vi "PicoScope6000aGetValuesOverlapped.vi"(5 "Segment Range":T1 {"toSegmentIndex" format="%.4p"; "fromSegmentIndex" format="%.4p"}, 7 "Buffer and Transfer Settings":T2 {"Down-Sample Mode" items=["None", "Aggregate", "Decimate", "Average"]; "Down Sample Ratio" step=1; "Samples" format="%_6p"}, 8 "error in (no error)":errorcluster, 11 "handle in":i16) -> (0 "error out":errorcluster, 3 "handle out":i16, 4 "overflow":i16[](array[numeric]) format="%10b", 6 "noOfSamples":u64)   [LabVIEW 2009]
doc: "Calls ps6000aGetValues"
uses:
  ps6000a.dll
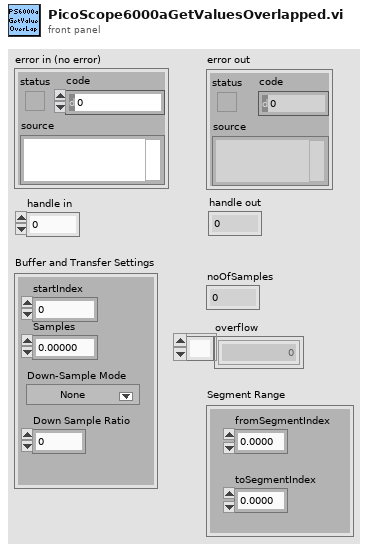
[diagram p1: front panel]
types:
  T1 = cluster{"fromSegmentIndex":u64, "toSegmentIndex":u64}
  T2 = cluster{"startIndex":u64, "Samples":u64, "Down Sample Ratio":u64, "Down-Sample Mode":u32}
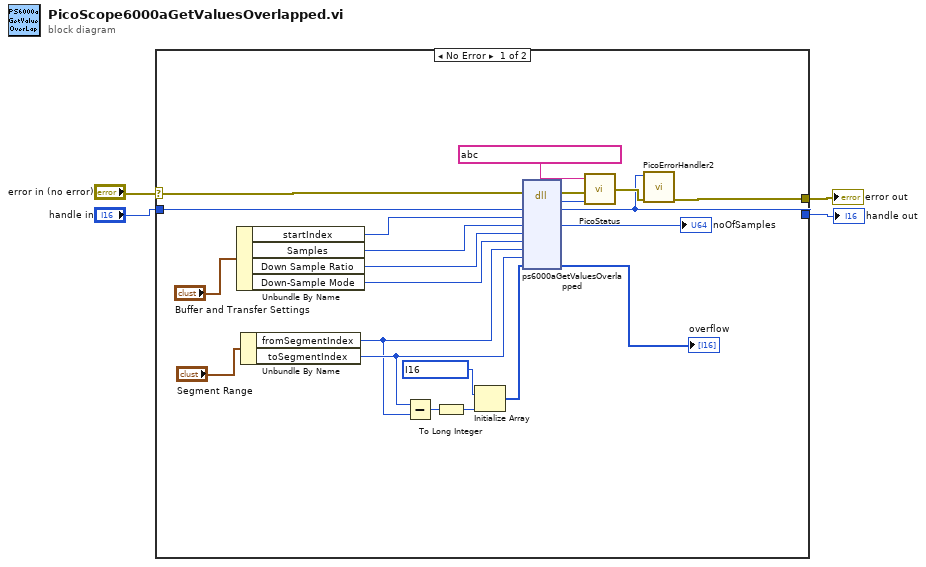
[diagram p0: block diagram]
diagram:
  n1 = case shown="No Error" "error in (no error)" {
    selector: "error in (no error)" -> [w17 w27]
    tunnel: "handle in" -> [w16 w28]
    tunnel: [w14 w28] -> w4
    tunnel: [w15 w27] -> w3
    frame #0 {
      n2 = Unbundle By Name("Buffer and Transfer Settings") -> ("startIndex"=w18:u64, "Samples"=w26:u64, "Down Sample Ratio"=w23:u64, "Down-Sample Mode"=w24:u32)
      n3 = Unbundle By Name("Segment Range") -> ("fromSegmentIndex"=w7:u64, "toSegmentIndex"=w8:u64)
      n4 = Subtract(x=w8, y=w7) -> (x-y=w6:u64)
      n5 = To Long Integer(number=w6) -> (32bit integer=w5:i32)
      n6 = Initialize Array(i16 ? ("overflow"), w5) -> (w10:i16[])
      n7 = dll-call lib="ps6000a.dll" fn="ps6000aGetValuesOverlapped" ("ps3000.dll:_ps3000_open_unit@0")(error in=w17, "handle"=w16, "startIndex"=w18, "noOfSamples"=w26, "downSampleRatio"=w23, "downSampleRatioMode"=w24, "fromSegmentIndex"=w7, "toSegmentIndex"=w8, "overflow"=w10) -> (error out=w22:errorcluster, "PICO_STATUS"=w21:u32, "handle"=w14:i16, "noOfSamples"=→"noOfSamples":u64, "overflow"=→"overflow":i16[])  [unwired: 7 in, 1 out]
      n8 = call "PicoStatus.vi"("PICO STATUS"=w21, "error in"=w22, "source"=string ?) -> ("error out"=w25:errorcluster)
      n9 = call "PicoErrorHandler2.vi"("error in (no error)"=w25, "handle In"=w14) -> ("error out"=w15:errorcluster)  [unwired: 9 in]
    }
    frame #1 {
    }
  }
  "error out" <- w3
  "handle out" <- w4
